vi "Pull_Data_via_Public_Server.vi"(3 "Path of File relative to EnFlo Data Root":path[](array[path])) -> (0 "error out":errorcluster, 1 "Relative Paths Out":path[](array[path]))   [LabVIEW 2012]
uses:
  Anemometry/Anemometry Sub Vis/Globals/Constants_global.vi
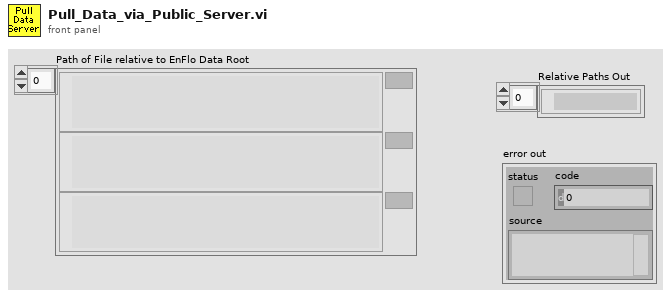
[diagram p1: front panel]
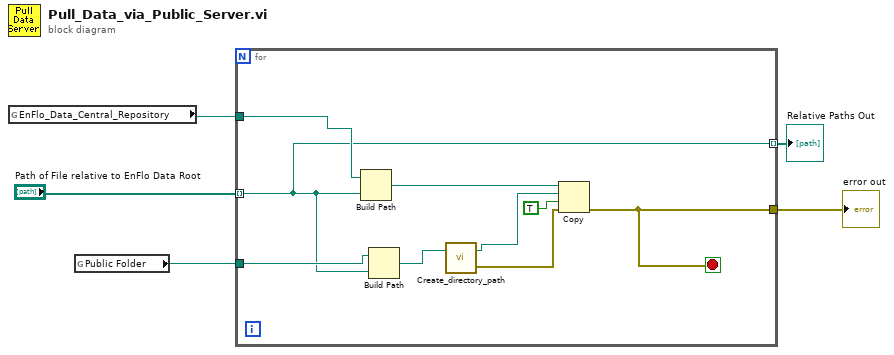
[diagram p0: block diagram]
diagram:
  n1 = global read "Constants_global.vi" "EnFlo_Data_Central_Repository"() -> (w5:path)
  n2 = global read "Constants_global.vi" "Public Folder"() -> (w2:path)
  n3 = for {
    tunnel: w5 -> [w14]
    tunnel: "Path of File relative to EnFlo Data Root" -> [w7] mode=indexing
    tunnel: w2 -> [w13]
    tunnel: [w8] -> w3
    tunnel: [w7] -> w1 mode=indexing
    stop <- w8 stop-if-true
    n4 = Build Path(base path=w14, name or relative path=w7) -> (appended path=w11:path)
    n5 = Build Path(base path=w13, name or relative path=w7) -> (appended path=w12:path)
    n6 = call "Create_directory_path.vi"("Path name"=w12) -> ("error out"=w9:errorcluster, "Path name Out"=w10:path)  [unwired: 1 in]
    n7 = Copy(8:w9, 9:TRUE ("overwrite (F)"), 10:w10, 11:w11) -> (0:w8:errorcluster)  [unwired: 1 in, 2 out]
  }
  "error out" <- w3
  "Relative Paths Out" <- w1
